vi "P4CMD Add.vi"(6 "keep checked out? (F)":bool, 7 "advanced options":variant, 8 "error in (no error)":errorcluster, 9 "comment":string, 10 "files":path[](array[path]), 11 "source control reference in":T1) -> (0 "error out":errorcluster, 1 "dialog box cancelled?":bool, 2 "status message":string, 3 "source control reference out":T1)   [LabVIEW 2017, in "NI_SCC_P4CMD.lvlib"]
uses:
  <vilib>/SourceControl/Providers/P4CMD/NI_SCC_P4CMD.lvlib
  <vilib>/SourceControl/sccapi/SCCAPI Refnum.ctl
  <vilib>/SourceControl/Providers/P4CMD/P4CMD Operations.ctl
  <vilib>/SourceControl/support/SCCSup Message Strings GLBL.vi
  <vilib>/SourceControl/sccapi/NI_SCC.lvlib
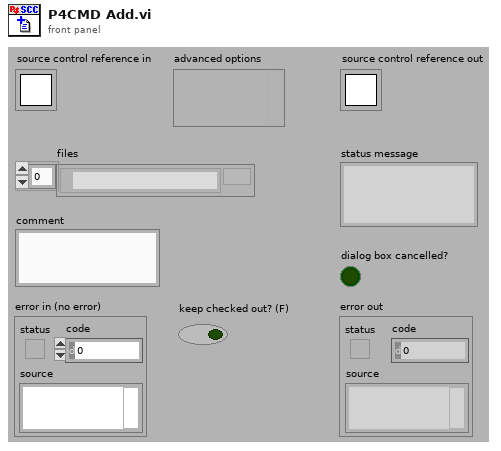
[diagram p1: front panel]
types:
  T1 = typedef "NI_SCC.lvlib/SCCAPI Refnum.ctl" = refnum<k1>
  T2 = typedef "NI_SCC_P4CMD.lvlib/P4CMD Operations.ctl" = enum16{"get all clients", "get all users", "describe changelist", "sync from depot", "open for edit", "submit to depot", "revert", "add to depot", "remove from depot", "print files revisions", "compare client file", "print depot file contents", "list opened files", "get file info", "lock files", "edit changelist spec", "info", "set variables"}
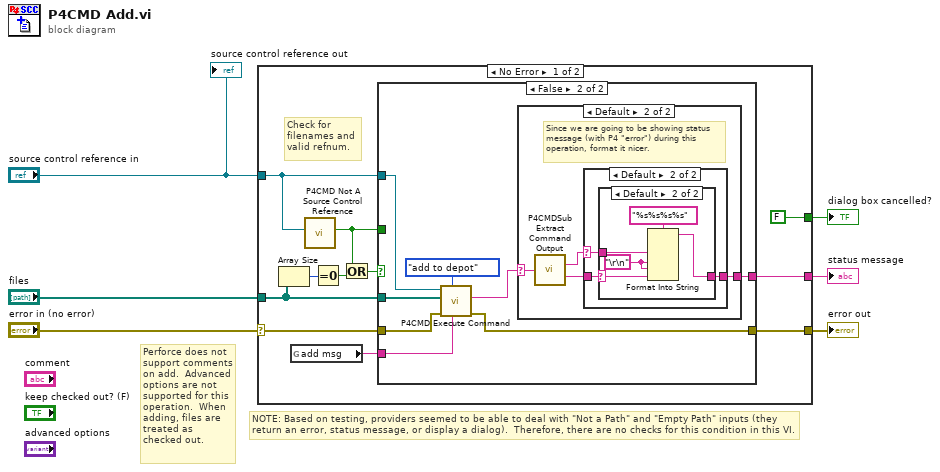
[diagram p0: block diagram]
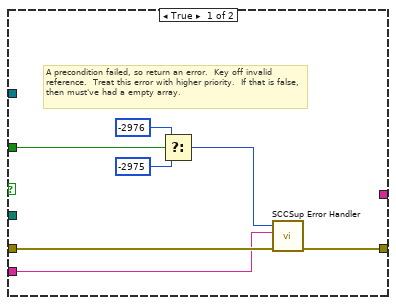
[diagram p2: hidden frame]
diagram:
  # "Perforce does not support comments on add.  Advanced options are not supported for this operation.  When adding, files are treated as checked out."
  # "NOTE: Based on testing, providers seemed to be able to deal with \"Not a Path\" and \"Empty Path\" inputs (they return an error, status message, or display a dialog).  Therefore, there are no checks for this condition in this VI."
  n1 = case shown="No Error" "error in (no error)" {
    selector: "error in (no error)" -> [w9 w48]
    tunnel: [w8 w48] -> w5
    tunnel: "source control reference in" -> [w14 _]
    tunnel: [w17 _] -> w3
    tunnel: "files" -> [w13 _]
    tunnel: [FALSE _] -> w1
    frame No Error {
      # "Check for filenames and valid refnum."
      n2 = Array Size(array=w13) -> (size(s)=w15:i32)
      n3 = global read "SCCSup Message Strings GLBL.vi" "add msg"() -> (w7:string)
      n4 = call <vilib>:"P4CMD Not A Source Control Reference.vi"("source control reference in"=w14) -> ("not a source control reference?"=w11:bool)  [unwired: 9 in, 1 out]
      n5 = Equal To 0?(x=w15) -> (x = 0?=w16:bool)
      n6 = Or(x=w11, y=w16) -> (x .or. y?=w12:bool)
      n7 = case shown="False" w12 {
        tunnel: w14 -> [_ w31]
        tunnel: [_ w26] -> w17
        tunnel: w13 -> [_ w30]
        tunnel: w11 -> [w22 _]
        tunnel: w9 -> [w20 w29]
        tunnel: [w19 w28] -> w8
        tunnel: w7 -> [w18 w27]
        frame True {
          # "A precondition failed, so return an error.  Key off invalid reference.  Treat this error with higher priority.  If that is false, then must've had a empty array."
          n8 = Select(t=-2976 ("result"), s=w22, f=-2975 ("result")) -> (s? t:f=w21:i32)
          n9 = call <vilib>:"SCCSup Error Handler.vi"("error in (no error)"=w20, "operation message"=w18, "scc error code"=w21) -> ("error out"=w19:errorcluster)  [unwired: 8 in]
        }
        frame False {
          n10 = call <vilib>:"P4CMD Execute Command.vi"("operation message"=w27, "p4 operation"=P4CMD_Operations."add to depot", "error in (no error)"=w29, "files"=w30, "source control reference in"=w31) -> ("error out"=w28:errorcluster, "command information"=w25:string)  [unwired: 4 in, 1 out]
          n11 = case shown="Default" w25 {
            selector: w25 -> [w33 w35]
            tunnel: [w33 w36] -> w26
            frame "" {
            }
            frame Default {
              # "Since we are going to be showing status message (with P4 \"error\") during this operation, format it nicer."
              n12 = call <vilib>:"P4CMDSub Extract Command Output.vi"("bundled message"=w35) -> ("command output"=w34:string, "command error"=w37:string)  [unwired: 13 in]
              n13 = case shown="Default" w34 {
                selector: w34 -> [_ w40]
                tunnel: w37 -> [w38 w39]
                tunnel: [w38 w41] -> w36
                frame "" {
                }
                frame Default {
                  n14 = case shown="Default" w39 {
                    selector: w39 -> [_ w43]
                    tunnel: [w42 w45] -> w41
                    tunnel: w40 -> [w42 w44]
                    frame "" {
                    }
                    frame Default {
                      w46 = "\r\n"
                      n15 = Format Into String(format string="%s%s%s%s", w44, w46, w46, w43) -> (resulting string=w45:string)  [unwired: 2 in, 1 out]
                    }
                  }
                }
              }
            }
          }
        }
      }
    }
    frame Error {
    }
  }
  "error out" <- w5
  "status message" <- w3
  "dialog box cancelled?" <- w1
  "source control reference out" <- "source control reference in"
